vi "SwitchACIR Channel UI.vi"() -> ()   [LabVIEW 2025, in "SwitchACIR Channel.lvclass"]
doc: "Copyright 2017 National Instruments Corporation\n\nLicensed under the Apache License, Version 2.0 (the \"License\"); you may not use this file except in compliance with the License. You may obtain a copy of the License at http://www.apache.org/licenses/LICENSE-2.0\nUnless required by applicable law or agreed to in writing, software distributed under the License is distributed on an \"AS IS\" BASIS, WITHOUT WARRANTIES OR CONDITIONS OF ANY KIND, either express or implied. See the License for the specific language governing permissions and limitations under the License."
uses:
  SwitchACIR Channel.lvclass
  SwitchACIR Channel.lvclass/SwitchACIR Channel.ctl
  Users/Public/Documents/Sandia National Labs/TSS Plugin/CEF.lvlibp/Node/CEF_Node.lvclass
  ACIR Instrument/ACIR Instrument.lvclass
  SwitchACIR Channel configuration/SwitchACIR Channel configuration.lvclass
  Users/Public/Documents/Sandia National Labs/TSS Plugin/CEF.lvlibp/Node/NodeRef.ctl
  Users/Public/Documents/Sandia National Labs/TSS Plugin/CEF.lvlibp/Node/UserEventRef.ctl
  Users/Public/Documents/Sandia National Labs/TSS Plugin/CEF.lvlibp/Node/mainQref.ctl
  Users/Public/Documents/Sandia National Labs/TSS Plugin/Abstract Engine.lvlibp/Channel configuration/Default Channel.ctl
  Users/Public/Documents/Sandia National Labs/TSS Plugin/Abstract Engine.lvlibp/Channel configuration/Channel configuration.lvclass
  SwitchACIR Channel configuration/SwitchACIR Channel Setting.ctl
panel:
  in  "SwitchACIR Channel":T3={"Default"={"Address"="localhost", "SW Alias"="ch0", "Enabled"=TRUE, "Type"="None", "Description"=""}, "SwitchACIR Channel Setting"={"Switch"=""}}
  in  "user event":T4
  in  "main queue":T5
  in  "node ref":T6
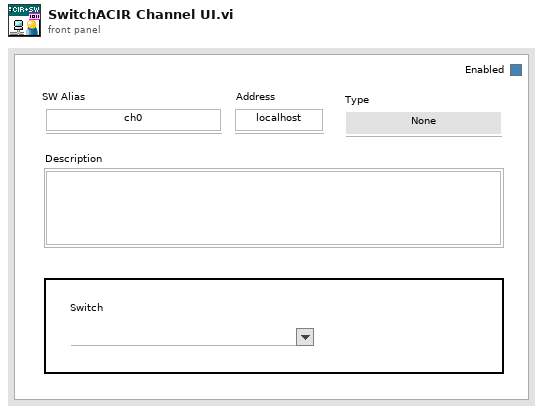
[diagram p1: front panel]
types:
  T1 = typedef "Abstract Engine.lvlibp/Channel configuration.lvclass/Default Channel.ctl" = cluster{"Address":string, "SW Alias":string, "Enabled":bool, "Type":string, "Description":string}
  T2 = typedef "SwitchACIR Channel configuration.lvclass/SwitchACIR Channel Setting.ctl" = cluster{"Switch":string}
  T3 = cluster{"Default":T1, "SwitchACIR Channel Setting":T2}
  T4 = typedef "CEF.lvlibp/CEF_Node.lvclass/UserEventRef.ctl" = refnum<user-event>
  T5 = typedef "CEF.lvlibp/CEF_Node.lvclass/mainQref.ctl" = refnum<queue>
  T6 = typedef "CEF.lvlibp/CEF_Node.lvclass/NodeRef.ctl" = refnum<data-value>
  T7 = cluster{"Channel Setting":T1, "SwitchACIR Channel":T2}
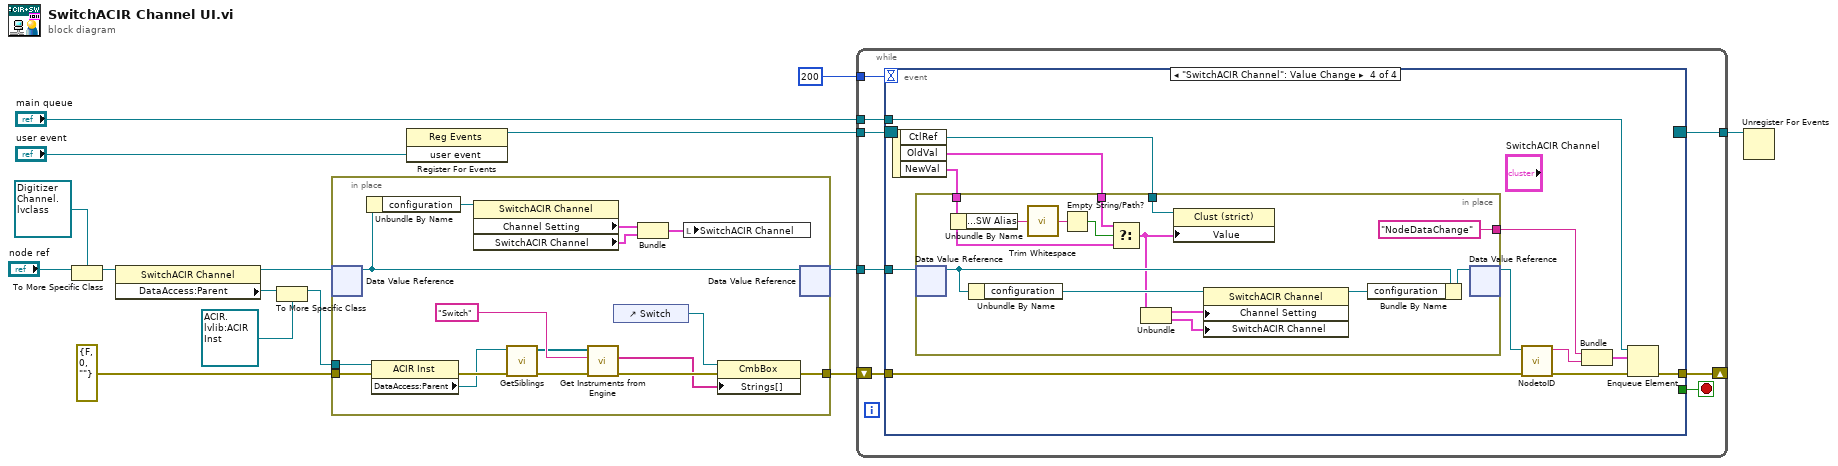
[diagram p0: block diagram]
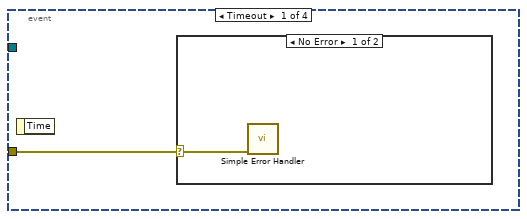
[diagram p2: hidden frame]
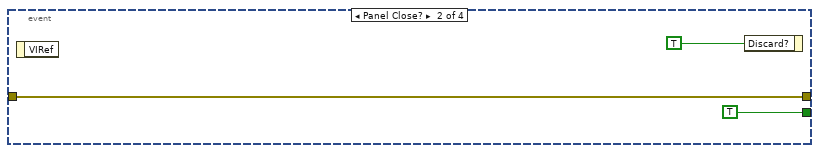
[diagram p4: hidden frame]
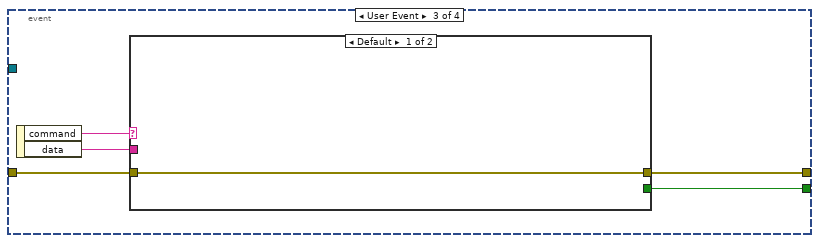
[diagram p5: hidden frame]
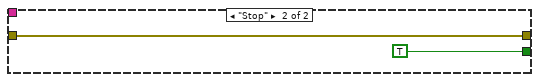
[diagram p6: hidden frame]
diagram:
  n1 = To More Specific Class(target class=refnum<data-value> refnum ("data value reference"), reference="node ref") -> (specific class reference=w10:refnum<data-value>)  [unwired: 1 in, 1 out]
  n2 = property class="SwitchACIR Channel"(reference=w10) -> (reference out=w6:refnum<data-value>, "DataAccess:Parent"=w5:refnum<data-value>)  [unwired: 1 in, 1 out]
  n3 = To More Specific Class(target class=refnum<data-value> refnum ("data value reference"), reference=w5) -> (specific class reference=w1:refnum<data-value>)  [unwired: 1 in, 1 out]
  n4 = in-place {
    in-place-border: errorcluster {"status"=FALSE, "code"=0, "source"=""} ("error out") -> [w21]
    in-place-border: [w26] -> w2
    in-place-border: w1 -> [w19]
    # "Initialize the front panel controls when loaded"
    n5 = in-place-dvr #1(w6) -> (w31:refnum<class "SwitchACIR Channel.lvclass">)  [unwired: 1 out]
    n6 = Unbundle By Name(w31) -> ("configuration"=w30:refnum<class "SwitchACIR Channel configuration.lvclass">)
    n7 = property class="ACIR Inst"(reference=w19, error in=w21) -> (error out=w20:errorcluster, "DataAccess:Parent"=w17:refnum<data-value>)  [unwired: 1 out]
    n8 = property class="SwitchACIR Channel"(reference=w30) -> ("Channel Setting"=w29:T1, "SwitchACIR Channel"=w28:T2)  [unwired: 1 in, 2 out]
    n9 = call "GetSiblings.vi"("error in"=w20, "node in"=w17) -> ("error out"=w18:errorcluster, "siblings"=w16:refnum<data-value>[])  [unwired: 8 in]
    n10 = call "Get Instruments from Engine.vi"("error in"=w18, "Engine"="Switch", "Engines"=w16) -> ("error out"=w23:errorcluster, "Instruments"=w22:string[])  [unwired: 6 in, 1 out]
    n11 = control-ref of="Switch"() -> (w25:refnum<vi>)
    n12 = Bundle("Channel Setting"=w29, "SwitchACIR Channel"=w28) -> (w27:T7)  [unwired: 1 in]
    n13 = local write "SwitchACIR Channel"(w27) -> ()
    n14 = property class="CmbBox"(reference=w25, error in=w23, "Strings[]"=w22) -> (error out=w26:errorcluster)  [unwired: 1 out]
    n15 = in-place-dvr #1(w31) -> (w9:refnum<data-value>)  [unwired: 1 out]
  }
  n16 = register-events("user event") -> (reference out=w14:refnum<event-registration>)  [unwired: 2 in, 1 out]
  n17 = while {
    tunnel: w9 -> [w39]
    tunnel: w14 -> [w38]
    tunnel: [w37] -> w13
    tunnel: "main queue" -> [w33]
    shift-right: [w34] -> _
    shift-left: w2 -> [w35]
    tunnel: 200 -> [w32]
    stop <- w36 stop-if-true
    n18 = event shown="[3] \"SwitchACIR Channel\": Value Change" {
      selector: w38 -> [_ _ _ _]
      dyn-events: [_ _ _ _] -> w37
      timeout: w32 -> [_ _ _ _]
      tunnel: w39 -> [_ _ _ w63]
      tunnel: [_ TRUE w49 _] -> w36
      tunnel: [_ w42 w45 w64] -> w34
      tunnel: w35 -> [w40 w42 w47 w54]
      tunnel: w33 -> [_ _ _ w58]
      event Timeout {
        n19 = event-data() -> ()  [unwired: 1 in, 1 out]
        n20 = case shown="No Error" w40 {
          selector: w40 -> [w41 _]
          frame No Error {
            n21 = call <vilib>:"Simple Error Handler.vi"("error in (no error)"=w41) -> ()  [unwired: 4 in, 5 out]
          }
          frame Error {
          }
        }
      }
      event Panel Close? {
        n22 = event-data() -> ()  [unwired: 1 in, 1 out]
        n23 = event-data("Discard?"=TRUE) -> ()  [unwired: 1 in, 1 out]
      }
      event User Event {
        n24 = event-data() -> ("command"=w46:string, "data"=w48:string)  [unwired: 1 in]
        n25 = case shown="Default" w46 {
          tunnel: [_ TRUE] -> w49
          tunnel: w48 -> [_ _]
          tunnel: w47 -> [w50 w51]
          tunnel: [w50 w51] -> w45
          frame Default {
          }
          frame "Stop" {
          }
        }
      }
      event "SwitchACIR Channel": Value Change {
        n26 = event-data() -> ("CtlRef"=w59:refnum<vi>, "OldVal"=w60:T3, "NewVal"=w61:T3)  [unwired: 1 in]
        n27 = in-place {
          in-place-border: w61 -> [w72]
          in-place-border: w60 -> [w75]
          in-place-border: w59 -> [w74]
          in-place-border: ["NodeDataChange" ("Message Name")] -> w56
          n28 = in-place-dvr #2(w63) -> (w78:refnum<class "SwitchACIR Channel.lvclass">)  [unwired: 1 out]
          n29 = Unbundle By Name(w72) -> ("Default.SW Alias"=w73:string)
          n30 = Unbundle By Name(w78) -> ("configuration"=w69:refnum<class "SwitchACIR Channel configuration.lvclass">)
          n31 = call <vilib>:"Trim Whitespace.vi"("string"=w73) -> ("trimmed string"=w70:string)  [unwired: 1 in]
          n32 = Empty String/Path?(string/path=w70) -> (empty?=w71:bool)
          n33 = Select(t=w75, s=w71, f=w72) -> (s? t:f=w67:T3)
          n34 = Unbundle(w67) -> ("Default"=w66:T1, "SwitchACIR Channel Setting"=w65:T2)
          n35 = property class="Clust (strict)"(reference=w74, "Value"=w67) -> ()  [unwired: 1 in, 2 out]
          n36 = property class="SwitchACIR Channel"(reference=w69, "Channel Setting"=w66, "SwitchACIR Channel"=w65) -> (reference out=w76:refnum<class "SwitchACIR Channel configuration.lvclass">)  [unwired: 1 in, 1 out]
          n37 = Bundle By Name(cluster=w78, "configuration"=w76) -> (w77:refnum<class "SwitchACIR Channel.lvclass">)
          n38 = in-place-dvr #2(w77) -> (w62:refnum<data-value>)  [unwired: 1 out]
        }
        n39 = call "NodetoID.vi"("error in"=w54, "node ref"=w62) -> ("error out"=w53:errorcluster, "ID"=w57:string)  [unwired: 8 in]
        n40 = Bundle("Message Name"=w56, "ID"=w57) -> (w55:cluster{"Message Name":string, "ID":string})  [unwired: 1 in]
        n41 = Enqueue Element(queue=w58, element=w55, error in (no error)=w53) -> (error out=w64:errorcluster)  [unwired: 1 in, 2 out]
      }
    }
  }
  n42 = Unregister For Events(event registration refnum=w13) -> ()  [unwired: 1 in, 1 out]
